vi "KepcoDCPwr Disable.vi"(0 "VISA Session":refnum<visa-resource-name>, 5 "Model In":string, 7 "channel name (\"\")":string="\"\"", 11 "error in (no error)":errorcluster {"code" format="%.0x"}) -> (4 "VISA Session Out":refnum<visa-resource-name>, 6 "Model Out":string, 8 "channel name out (\"\")":string="\"\"" caption="channel name Out (\"\")", 15 "error out":errorcluster {"code" format="%.0x"})   [LabVIEW 2010]
doc: "This VI places the instrument in a quiescent state where it has minimal or no impact on the system to which it is connected."
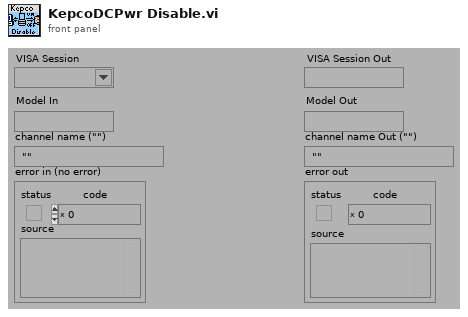
[diagram p1: front panel]
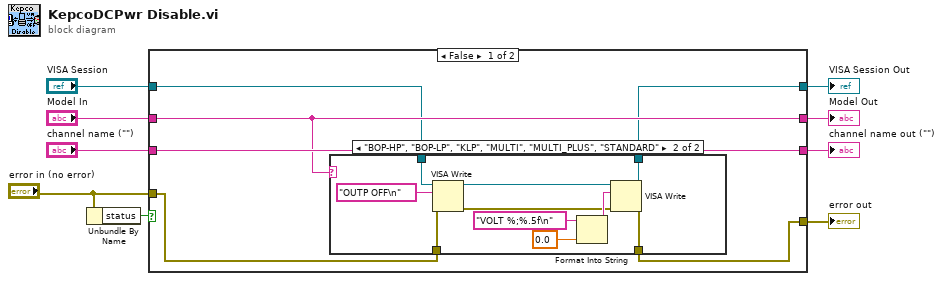
[diagram p0: block diagram]
diagram:
  n1 = Unbundle By Name("error in (no error)") -> ("status"=w8:bool)
  n2 = case shown="False" w8 {
    tunnel: [w11 w31] -> w9
    tunnel: "error in (no error)" -> [w10 w31]
    tunnel: "VISA Session" -> [w13 w30]
    tunnel: "Model In" -> [w14 w29]
    tunnel: "channel name (\"\")" -> [w15 w28]
    tunnel: [w12 w30] -> w3
    tunnel: [w14 w29] -> w2
    tunnel: [w15 w28] -> w1
    frame False {
      n3 = case shown="\"BOP-HP\", \"BOP-LP\", \"KLP\", \"MULTI\", \"MULTI_PLUS\", \"STANDARD\"" w14 {
        tunnel: w13 -> [w16 w23]
        tunnel: w10 -> [w17 w22]
        tunnel: [w16 w21] -> w12
        tunnel: [w17 w20] -> w11
        frame "", Default {
        }
        frame "BOP-HP", "BOP-LP", "KLP", "MULTI", "MULTI_PLUS", "STANDARD" {
          n4 = VISA Write(VISA resource name=w23, write buffer="OUTP OFF\n", error in (no error)=w22) -> (VISA resource name out=w18:refnum<visa-resource-name>, error out=w19:errorcluster)  [unwired: 1 out]
          n5 = Format Into String(format string="VOLT %;%.5f\n", 0.0 ("level (0.0 volts)")) -> (resulting string=w24:string)  [unwired: 2 in, 1 out]
          n6 = VISA Write(VISA resource name=w18, write buffer=w24, error in (no error)=w19) -> (VISA resource name out=w21:refnum<visa-resource-name>, error out=w20:errorcluster)  [unwired: 1 out]
        }
      }
    }
    frame True {
    }
  }
  "error out" <- w9
  "channel name out (\"\")" <- w1
  "Model Out" <- w2
  "VISA Session Out" <- w3
